vi "AD5781SetGlobalVariables.vi"   [LabVIEW 2014]
uses:
  Controls/FPGA SPI_FPGA SPI State.ctl
  <vilib>/rvi/Emulation/niFpgaSctlEmulationGetInTimedLoop.vi
  Code/FPGA SPI_Globals.vi
  <vilib>/rvi/Emulation/niFpgaProcessEmulError.vi
types:
  T1 = typedef "FPGA SPI_FPGA SPI State.ctl" = enum8{"Idle", "Read/Write SPI", "Configure"}
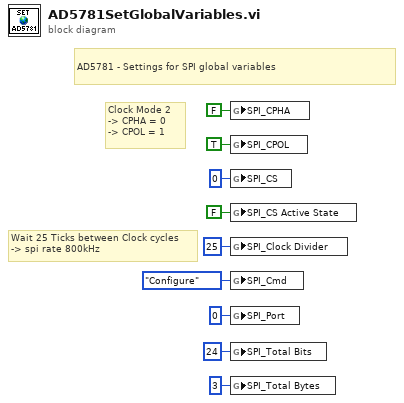
[diagram p0: block diagram]
diagram:
  # "AD5781 - Settings for SPI global variables"
  # "Clock Mode 2 \n-> CPHA = 0\n-> CPOL = 1"
  # "Wait 25 Ticks between Clock cycles\n-> spi rate 800kHz"
  n1 = global write "FPGA SPI_Globals.vi" "SPI_CPHA"(FALSE ("SPI_CPHA")) -> ()
  n2 = global write "FPGA SPI_Globals.vi" "SPI_CPOL"(TRUE ("SPI_CPOL")) -> ()
  n3 = global write "FPGA SPI_Globals.vi" "SPI_CS"(u8 0 ("SPI_CS")) -> ()
  n4 = global write "FPGA SPI_Globals.vi" "SPI_CS Active State"(FALSE ("SPI_CS Active State")) -> ()
  n5 = global write "FPGA SPI_Globals.vi" "SPI_Clock Divider"(u32 25 ("SPI_Clock Divider")) -> ()
  n6 = global write "FPGA SPI_Globals.vi" "SPI_Cmd"(FPGA_SPI_FPGA_SPI_State."Configure" ("SPI_Cmd")) -> ()
  n7 = global write "FPGA SPI_Globals.vi" "SPI_Port"(i8 0 ("SPI_Port")) -> ()
  n8 = global write "FPGA SPI_Globals.vi" "SPI_Total Bits"(u16 24 ("SPI_Total Bits")) -> ()
  n9 = global write "FPGA SPI_Globals.vi" "SPI_Total Bytes"(u16 3 ("SPI_Total Bytes")) -> ()
